vi "Replace Single Wheel in Steering Frame by Name.vi"(5 "x position":dbl, 6 "frame angle (rad)":dbl=nan, 7 "y position":dbl, 8 "error in (no error)":errorcluster, 9 "wheel":refnum<class "NI_Robotics_Wheel.lvclass">, 10 "wheel name":string, 11 "steering frame in":refnum<class "NI_Robotics_Steering Frame.lvclass">) -> (0 "error out":errorcluster, 1 "found?":bool, 3 "steering frame out":refnum<class "NI_Robotics_Steering Frame.lvclass">)   [LabVIEW 2017, in "NI_Robotics_Steering Frame.lvclass"]
doc: "Replaces wheels in <B>steering frame in</B> with the wheels you specify. You must manually select the polymorphic instance to use."
uses:
  <vilib>/robotics/Steering/Steering Frame/NI_Robotics_Steering Frame.lvclass
  <vilib>/robotics/Steering/Wheel/NI_Robotics_Wheel.lvclass
  <vilib>/robotics/Steering/Steering Frame/NI_Robotics_Steering Frame.lvclass/NI_Robotics_Steering Frame.ctl
  <vilib>/robotics/Steering/Wheel/NI_Robotics_Wheel.lvclass/NI_Robotics_Wheel.ctl
  <vilib>/robotics/Steering/Steering Frame/Get Indexes of Multiple Wheels from Names.vi
  <vilib>/robotics/Steering/Wheel/Get Wheel Name.vi
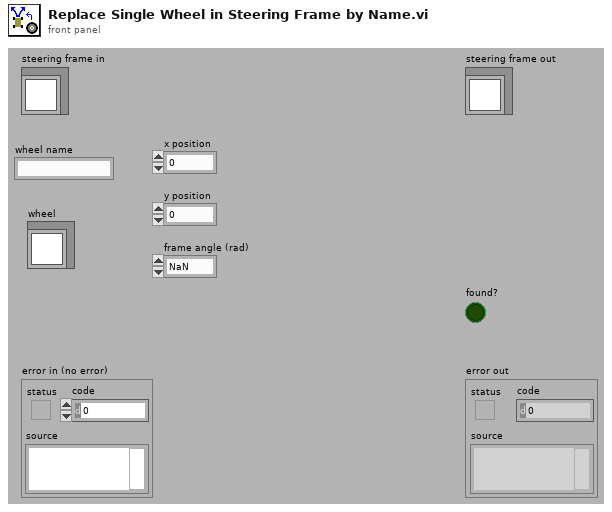
[diagram p1: front panel]
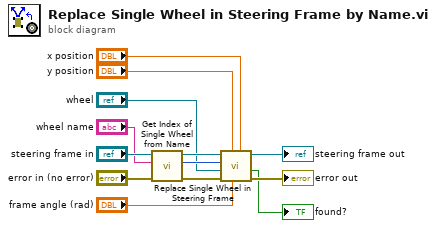
[diagram p0: block diagram]
diagram:
  n1 = call <vilib>:"Get Index of Single Wheel from Name.vi"("error in (no error)"="error in (no error)", "wheel name"="wheel name", "steering frame in"="steering frame in") -> ("error out"=w8:errorcluster, "index"=w9:i32, "steering frame out"=w10:refnum<class "NI_Robotics_Steering Frame.lvclass">)  [unwired: 5 in, 1 out]
  n2 = call <vilib>:"Replace Single Wheel in Steering Frame.vi"("x position"="x position", "frame angle (rad)"="frame angle (rad)", "y position"="y position", "error in (no error)"=w8, "wheel"="wheel", "wheel index"=w9, "steering frame in"=w10) -> ("error out"=→"error out":errorcluster, "found?"=→"found?":bool, "steering frame out"=→"steering frame out":refnum<class "NI_Robotics_Steering Frame.lvclass">)  [unwired: 2 in]
